vi "Image Size.vi"(4 "Error":string, 7 "Image":T1={"Image ID"=0, "Channel ID"=-1}) -> (0 "Error":string, 1 "Height":i32, 2 "Width":i32, 3 "Image":T1={"Image ID"=0, "Channel ID"=-1})   [LabVIEW 2011, in "labvvis.lvlib"]
doc: "Returns the width and height of a LabVVIS image."
uses:
  <userlib>/labvvis/labvvis.lvlib
  <userlib>/labvvis/VVIS Image.ctl
  labvvis.framework
panel:
  in  "Height":i32
  in  "Width":i32
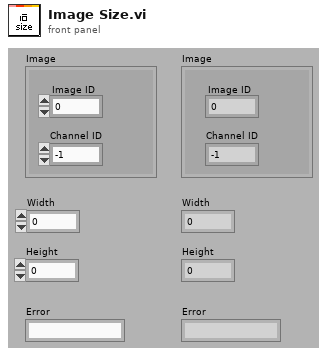
[diagram p1: front panel]
types:
  T1 = typedef "labvvis.lvlib/VVIS Image.ctl" = cluster{"Image ID":i16, "Channel ID":i16}
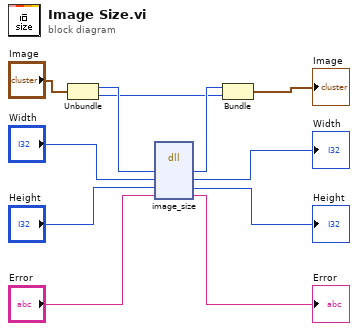
[diagram p0: block diagram]
diagram:
  n1 = Unbundle("Image") -> ("Image ID"=w9:i16, "Channel ID"=w1:i16)
  n2 = dll-call lib="labvvis.framework" fn="image_size"("out"=w9, "width"="Width", "height"="Height", "error"="Error") -> ("out"=w8:i16, "width"=→"Width":i32, "height"=→"Height":i32, "error"=→"Error":string)  [unwired: 4 in, 2 out]
  n3 = Bundle("out"=w8, "Channel ID"=w1) -> (→"Image":cluster{"out":i16, "Channel ID":i16})  [unwired: 1 in]
